vi "Toggle Descendants.vi"(8 "error in (no error)":errorcluster, 10 "Tag":string, 11 "TreeHier in":refnum<class "TreeSelectionHierarchal.lvclass">) -> (0 "error out":errorcluster, 3 "TreeHier out":refnum<class "TreeSelectionHierarchal.lvclass">)   [LabVIEW 2015, in "TreeSelectionHierarchal.lvclass"]
doc: "<b> </b> <b> </b>\n©2016 Q Software Innovations, LLC (QSI)\nwritten by Quentin Alldredge\nproduced in LabVIEW 2015\n\nsupport@qsoftwareinnovations.com\nwww.qsoftwareinnovations.com\n\nAll rights reserved.\n\nRedistribution and use in source and binary forms, with or without modification, are permitted provided that the following conditions are met:\n\n * Redistributions of source code must retain the above copyright notice, this list of conditions and the following disclaimer.\n * Redistributions in binary form must reproduce the above copyright notice, this list of conditions and the following disclaimer in the documentation and/or other materials provided with the distribution.\n * Neither the name of Q Software Innovations, LLC. nor the names of its contributors may be used to endorse or promote products derived from this software without specific prior written permission.\n\nTHIS SOFTWARE IS PROVIDED BY THE COPYRIGHT HOLDERS AND CONTRIBUTORS \"AS IS\" AND ANY EXPRESS OR IMPLIED WARRANTIES, INCLUDING, BUT NOT LIMITED TO, THE IMPLIED WARRANTIES OF MERCHANTABILITY AND FITNESS FOR A PARTICULAR PURPOSE ARE DISCLAIMED. IN NO EVENT SHALL THE COPYRIGHT OWNER OR CONTRIBUTORS BE LIABLE FOR ANY DIRECT, INDIRECT, INCIDENTAL, SPECIAL, EXEMPLARY, OR CONSEQUENTIAL DAMAGES (INCLUDING, BUT NOT LIMITED TO, PROCUREMENT OF SUBSTITUTE GOODS OR SERVICES; LOSS OF USE, DATA, OR PROFITS; OR BUSINESS INTERRUPTION) HOWEVER CAUSED AND ON ANY THEORY OF LIABILITY, WHETHER IN CONTRACT, STRICT LIABILITY, OR TORT (INCLUDING NEGLIGENCE OR OTHERWISE) ARISING IN ANY WAY OUT OF THE USE OF THIS SOFTWARE, EVEN IF ADVISED OF THE POSSIBILITY OF SUCH DAMAGE."
uses:
  TreeSelectionHierarchal.lvclass
  TreeControl/TreeControl.lvclass
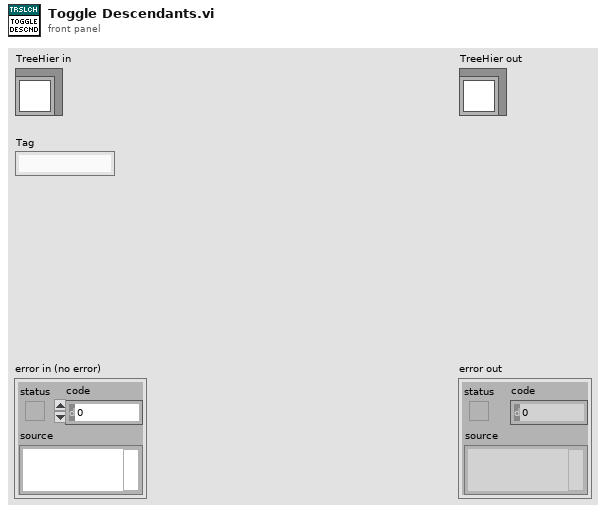
[diagram p1: front panel]
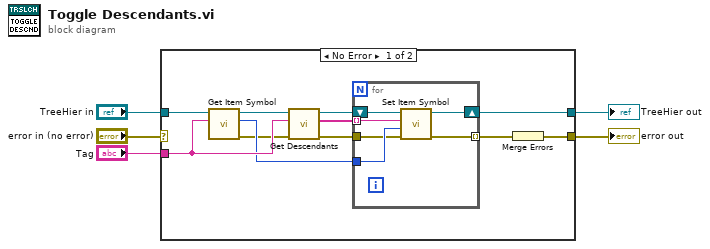
[diagram p0: block diagram]
diagram:
  n1 = case shown="No Error" "error in (no error)" {
    selector: "error in (no error)" -> [_ w24]
    tunnel: [w6 w24] -> w4
    tunnel: [w16 w23] -> w2
    tunnel: "TreeHier in" -> [w13 w23]
    tunnel: "Tag" -> [w11 _]
    frame No Error {
      n2 = call "Get Item Symbol.vi"("Tag"=w11, "Tree in"=w13) -> ("error out"=w9:errorcluster, "Symbol Index"=w10:i32, "Tree out"=w12:refnum<class "TreeSelectionHierarchal.lvclass">)  [unwired: 7 in]
      n3 = call "Get Descendants.vi"("error in (no error)"=w9, "Tag"=w11, "Tree in"=w12) -> ("error out"=w8:errorcluster, "DescendantTags[]"=w14:string[], "Tree out"=w15:refnum<class "TreeSelectionHierarchal.lvclass">)  [unwired: 6 in]
      n4 = for {
        shift-right: [w21] -> w16
        shift-left: w15 -> [w22]
        tunnel: w14 -> [w20] mode=indexing
        tunnel: w10 -> [w19]
        tunnel: w8 -> [w18]
        tunnel: [w17] -> w7 mode=indexing
        n5 = call "Set Item Symbol.vi"("error in (no error)"=w18, "Symbol Index"=w19, "Tag"=w20, "Tree in"=w22) -> ("error out"=w17:errorcluster, "Tree (dup)"=w21:refnum<class "TreeSelectionHierarchal.lvclass">)  [unwired: 6 in]
      }
      n6 = Merge Errors(w7) -> (w6:errorcluster)
    }
    frame Error {
    }
  }
  "error out" <- w4
  "TreeHier out" <- w2
